vi "TPNT_GetID.vi"(7 "device":string, 9 "index in":i32, 10 "testpoint In":T1={"name"="", "type"="", "algor"=[], "update_rate"=0.0, "Limits"={"Alarm Type"="", "Lower "=0.0, "Upper"=0.0, "Nominal"=0.0, "outrange"=FALSE, "Check"=TRUE, "latch"=FALSE, "level"=""}, "Samples"={"samples"=0, "counter"=0, "Values"=[], "Current Value"="", "filter"="", "precision"=2}, "next_update"=0, "Status"="", "monitor"=TRUE, "error"=FALSE, "Log"={"log"=FALSE, "file"=path "", "type"="", "format"="", "updaterate"=0.0, "nex_update"=0, "mode"=""}, "permissions"="", "ID"=""} {"Log"."updaterate" format="%.2f"; "Samples"."Values" format="%.2f"; "Samples"."samples" min=1 step=1; "Limits"."Nominal" format="%.2f"; "Limits"."Upper" format="%.2f"; "Limits"."Lower" format="%.2f"; "update_rate" format="%.2f"}) -> (1 "id out":string, 2 "id?":bool)   [LabVIEW 2016]
uses:
  TPNT_TP.ctl
  TPNT_Limits.ctl
  TPNT_Samples.ctl
  TPNT_Log.ctl
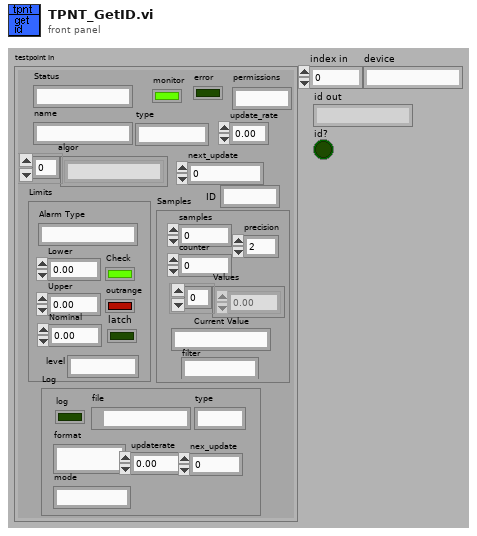
[diagram p1: front panel]
types:
  T1 = typedef "TPNT_TP.ctl" = cluster{"name":string, "type":string, "algor":string[], "update_rate":sgl, "Limits":T2, "Samples":T3, "next_update":u32, "Status":string, "monitor":bool, "error":bool, "Log":T4, "permissions":string, "ID":string}
  T2 = typedef "TPNT_Limits.ctl" = cluster{"Alarm Type":string, "Lower ":dbl, "Upper":dbl, "Nominal":dbl, "outrange":bool, "Check":bool, "latch":bool, "level":string}
  T3 = typedef "TPNT_Samples.ctl" = cluster{"samples":i32, "counter":i32, "Values":dbl[], "Current Value":string, "filter":string, "precision":u8}
  T4 = typedef "TPNT_Log.ctl" = cluster{"log":bool, "file":path, "type":string, "format":string, "updaterate":dbl, "nex_update":u32, "mode":string}
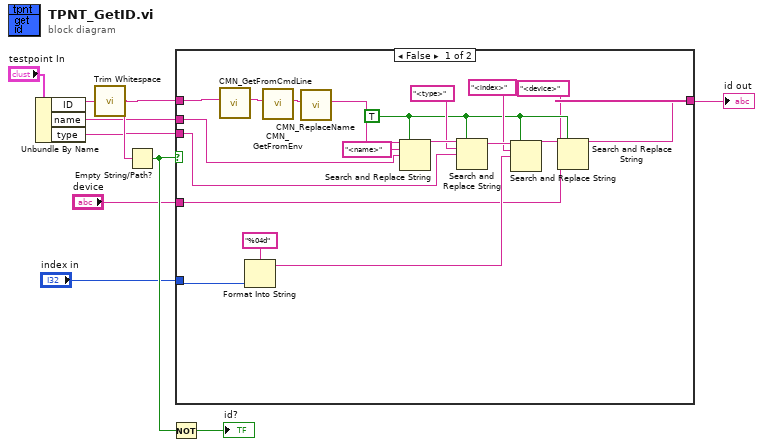
[diagram p0: block diagram]
diagram:
  n1 = Unbundle By Name("testpoint In") -> ("ID"=w5:string, "name"=w4:string, "type"=w3:string)
  n2 = call <vilib>:"Trim Whitespace.vi"("string"=w5) -> ("trimmed string"=w10:string)  [unwired: 1 in]
  n3 = Empty String/Path?(string/path=w10) -> (empty?=w9:bool)
  n4 = Not(x=w9) -> (.not. x?=→"id?":bool)
  n5 = case shown="False" w9 {
    tunnel: w10 -> [w27 w30]
    tunnel: [w12 w30] -> w8
    tunnel: w4 -> [w24 _]
    tunnel: w3 -> [w21 _]
    tunnel: "index in" -> [w18 _]
    tunnel: "device" -> [w11 _]
    frame False {
      w14 = TRUE ("replace all? (F)")
      n6 = call "CMN_GetFromCmdLine.vi"("str in"=w27) -> ("str out"=w29:string)  [unwired: 10 out]
      n7 = Format Into String(format string="%04d", w18) -> (resulting string=w16:string)  [unwired: 2 in, 1 out]
      n8 = call "CMN_GetFromEnv.vi"("str in"=w29) -> ("str out"=w28:string)  [unwired: 10 out]
      n9 = call "CMN_ReplaceName.vi"("name in"=w28) -> ("name out"=w26:string)  [unwired: 1 in, 9 out]
      n10 = Search and Replace String(replace all?=w14, input string=w26, search string="<name>", replace string=w24) -> (result string=w23:string)  [unwired: 1 in, 6 out]
      n11 = Search and Replace String(replace all?=w14, input string=w23, search string="<type>", replace string=w21) -> (result string=w20:string)  [unwired: 1 in, 6 out]
      n12 = Search and Replace String(replace all?=w14, input string=w20, search string="<index>", replace string=w16) -> (result string=w15:string)  [unwired: 1 in, 6 out]
      n13 = Search and Replace String(replace all?=w14, input string=w15, search string="<device>", replace string=w11) -> (result string=w12:string)  [unwired: 1 in, 6 out]
    }
    frame True {
    }
  }
  "id out" <- w8
